vi "PCO_InitDSNUAdjustment.vi"(0 "ph":u64, 7 "wDSNUAdjustMode":u16(ring) items=["No DSNU Correction", "Auto DSNU Correction", "Manual DSNU Correction"], 11 "error in (no error)":errorcluster {"code" format="%x"}) -> (4 "ph out":u64, 6 "ErrorMessage":i32 format="%x", 15 "error out":errorcluster {"code" format="%x"})   [LabVIEW 2019, in "SDK.lvlib" / "ImageSensor.lvlib"]
doc: "Initiates the DSNU correction in manual DSNU adjustment mode"
uses:
  ImageSensor.lvlib
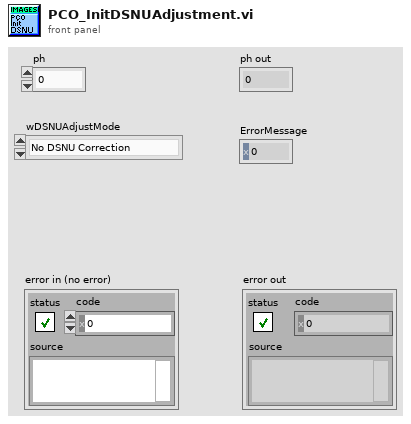
[diagram p1: front panel]
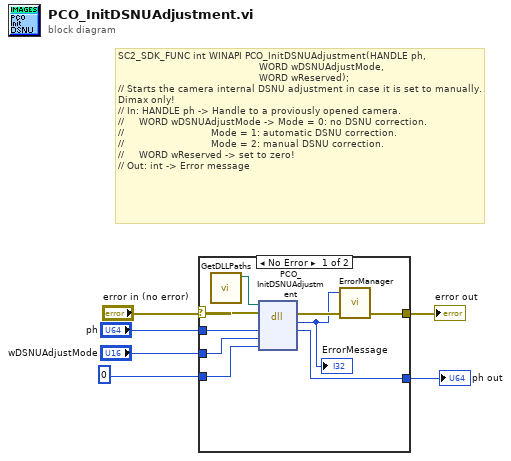
[diagram p0: block diagram]
diagram:
  # "SC2_SDK_FUNC int WINAPI PCO_InitDSNUAdjustment(HANDLE ph,\n                                               WORD wDSNUAdjustMode,\n                                               WORD wReserved);\n// Starts the camera internal DSNU adjustment in case it is set to manually. Dimax only!\n// In: HANDLE ph -> Handle to a proviously opened camera.\n//     WORD wDSNUAdjustMode -> Mode = 0: no DSNU correction.\n//                             Mode = 1: automatic DSNU correction.\n//                             Mode = 2: manual DSNU correction.\n//     WORD wReserved -> set to zero!\n// Out: int -> Error message"
  n1 = case shown="No Error" "error in (no error)" {
    selector: "error in (no error)" -> [w10 w17]
    tunnel: "ph" -> [w15 w16]
    tunnel: [w14 w16] -> w5
    tunnel: [w12 w17] -> w4
    tunnel: "wDSNUAdjustMode" -> [w8 _]
    tunnel: u16 0 ("wReserved") -> [w7 _]
    frame No Error {
      n2 = call "GetDLLPaths.vi"() -> ("SC2_Cam_Path"=w9:path)  [unwired: 8 in, 3 out]
      n3 = dll-call lib="?" fn="PCO_InitDSNUAdjustment"(path in=w9, error in=w10, "ph"=w15, "wDSNUAdjustMode"=w8, "wReserved"=w7) -> (error out=w13:errorcluster, "return type"=w11:i32, "ph"=w14:u64)  [unwired: 3 in, 1 out]
      "ErrorMessage" <- w11
      n4 = call "ErrorManager.vi"("error in (no error)"=w13, "error code"=w11) -> ("error out"=w12:errorcluster)  [unwired: 2 in, 1 out]
    }
    frame Error {
    }
  }
  "ph out" <- w5
  "error out" <- w4
